vi "VisualizeCHROMAOUT.vi"() -> ()   [LabVIEW 2018, in "Visualization.lvlib" / "VisualizeAcPwr.lvclass"]
doc: "This VI listens for any measurement data associated with the provided PluginName and displays it to the user for analysis. The display is only suitable for data coming from the Chroma Plugin."
uses:
  VisualizeAcPwr.lvclass
  VisualizeBase/VisualizeBase_class/Requests/VisUserEventType.ctl
  <vilib>/event_ctls.llb/usereventprio.ctl
  AcPwr/AcPwrShared/clMeasurmentData.ctl
  <extravilib>/ChannelInstances/Tag-bool/Read With Abort.vi
  <extravilib>/ChannelInstances/Tag-bool/Write With Abort.vi
  <extravilib>/ChannelInstances/Tag-bool/Instantiate.vi
  <extravilib>/ChannelInstances/Tag-bool/EndpointRead.vi
  <vilib>/Utility/error.llb/Error Cluster From Error Code.vi
  <extravilib>/ChannelInstances/Tag-bool/Endpoint.vi
  <vilib>/ErrorRing/Error Ring.xnode
  VisualizeBase/VisualizeBase_class/VisualizeBase.lvclass
  <userlib>/NIST/NISTErrorLib/NISTErrorLib.lvlib
  AcPwr/AcPwrShared/AcPwrShared.lvlib
  <extravilib>/ChannelInstances/Tag-bool.lvlib
panel:
  in  "Tab Control":enum32{"Chart", "XY Graph"}(tab)
  out "ChromaOutput":waveform(dbl)[](graph)=[{"t0"=timestamp(3657200531.6397257 s since 1904-01-01), "dt"=1.0, "Y"=[46.19]}, {"t0"=timestamp(3657200531.6397257 s since 1904-01-01), "dt"=1.0, "Y"=[2.0]}, {"t0"=timestamp(3657200531.6397257 s since 1904-01-01), "dt"=1.0, "Y"=[60.0]}]
  in  "PlotYAxis":u32[](array[numeric])=[0, 1, 0] max=1
  out "Incorrect DataType?":bool
  out "Chroma's Internal Errors/Warnings":string="No Error"
  out "Current (A)":dbl(knob) scale=0.0..15.0
  out "Voltage (V)":dbl(knob) scale=0.0..100.0
  out "XY Graph":cluster{dbl[], dbl[]}(graph)={[0.02, 0.02, 0.02, 0.02, 0.02, 0.02, 0.02, 0.02, 0.1, 0.1, 0.1, 0.1, 0.1, 0.11, 0.2, 0.2, 0.2, 0.2, 0.2, 0.2, 0.3, 0.3, 0.3, 0.3, 0.3, 0.3, 0.3, 0.37, 0.4, 0.4, 0.4, 0.4, 0.4, 0.4, 0.48, 0.5, 0.5, 0.5, 0.5, 0.5, 0.5, 0.59, 0.6, 0.6, 0.6, 0.6, 0.6, 0.6, 0.6, 0.69, 0.69, 0.69, 0.69, 0.69, 0.69, 0.71, 0.79, 0.79, 0.79, 0.79, 0.79, 0.79, 0.89, 0.89, 0.89, 0.89, 0.89, 0.89, 0.89, 1.0, 1.0, 1.0, 1.0, 1.0, 1.0, 1.0, 1.1, 1.1, 1.1, 1.09, 1.09, 1.09, 1.1, 1.19, 1.19, 1.2, 1.2, 1.2, 1.2, 1.2, 1.29, 1.29, 1.29, 1.29, 1.29, 1.29, 1.29, 1.39, 1.39, 1.39, 1.39, 1.39, 1.39, 1.39, 1.4, 1.49, 1.49, 1.49, 1.49, 1.49, 1.49, 1.57, 1.59, 1.59, 1.59, 1.59, 1.59, 1.59, 1.69, 1.69, 1.69, 1.69, 1.69, 1.69, 1.69, 1.79, 1.79, 1.79, 1.79, 1.79, 1.79, 1.79, 1.89, 1.89, 1.89, 1.89, 1.89, 1.89, 1.89, 1.99, 1.99, 1.99, 1.99, 1.99, 1.99, 2.0, 2.09, 2.09, 2.09, 2.09, 2.09, 2.09, 2.13, 2.19, 2.19, 2.19, 2.19, 2.19, 2.19, 2.29, 2.29, 2.29, 2.29, 2.29, 2.29, 2.29, 2.29, 2.39, 2.39, 2.39, 2.39, 2.39, 2.39, 2.39, 2.49, 2.49, 2.49, 2.49, 2.49, 2.49, 2.51, 2.59, 2.59, 2.59, 2.59, 2.59, 2.59, 2.69, 2.69, 2.69, 2.69, 2.69, 2.69, 2.69, 2.79, 2.79, 2.79, 2.79, 2.79, 2.79, 2.79, 2.81, 2.89, 2.89, 2.89, 2.89, 2.89, 2.89, 2.89, 2.99, 2.99, 2.99, 2.99, 2.99, 2.99, 3.0, 3.09, 3.09, 3.09, 3.09, 3.09, 3.09, 3.1, 3.19, 3.19, 3.19, 3.19, 3.19, 3.19, 3.29, 3.29, 3.29, 3.29, 3.29, 3.29, 3.29, 3.39, 3.39, 3.39, 3.39, 3.39, 3.39, 3.39, 3.39, 3.49, 3.49, 3.49, 3.49, 3.49, 3.49, 3.49, 3.5, 3.59, 3.59, 3.59, 3.59, 3.59, 3.59, 3.6, 3.69, 3.69, 3.69, 3.69, 3.69, 3.69, 3.79, 3.79, 3.79, 3.79, 3.79, 3.79, 3.79, 3.89, 3.89, 3.89, 3.89, 3.89, 3.89, 3.89, 3.99, 3.99, 3.99, 3.99, 3.99, 3.99, 3.99], [42.02, 41.83, 42.15, 41.98, 41.52, 41.47, 41.64, 41.55, 41.51, 41.49, 41.46, 41.51, 41.41, 41.39, 41.42, 41.42, 41.41, 41.4, 41.29, 41.3, 41.32, 41.33, 41.32, 41.31, 41.32, 41.21, 41.21, 41.2, 41.2, 41.21, 41.22, 41.21, 41.1, 41.1, 41.09, 41.1, 41.09, 41.11, 41.1, 40.98, 40.99, 40.98, 40.98, 40.99, 40.99, 40.98, 40.98, 40.86, 40.86, 40.88, 40.87, 40.88, 40.87, 40.87, 40.74, 40.75, 40.75, 40.75, 40.73, 40.76, 40.63, 40.63, 40.62, 40.64, 40.64, 40.61, 40.64, 40.6, 40.5, 40.46, 40.5, 40.51, 40.5, 40.51, 40.37, 40.37, 40.37, 40.37, 40.37, 40.38, 40.37, 40.36, 40.22, 40.23, 40.23, 40.24, 40.23, 40.24, 40.1, 40.09, 40.07, 40.11, 40.09, 40.09, 40.11, 39.96, 39.96, 39.95, 39.96, 39.96, 39.96, 39.94, 39.81, 39.79, 39.79, 39.81, 39.8, 39.79, 39.79, 39.81, 39.65, 39.65, 39.65, 39.65, 39.64, 39.64, 39.65, 39.48, 39.48, 39.48, 39.48, 39.47, 39.48, 39.31, 39.31, 39.3, 39.31, 39.32, 39.31, 39.31, 39.14, 39.13, 39.13, 39.14, 39.13, 39.14, 39.13, 38.95, 38.95, 38.95, 38.94, 38.95, 38.95, 38.95, 38.75, 38.75, 38.76, 38.76, 38.75, 38.75, 38.75, 38.56, 38.56, 38.56, 38.56, 38.56, 38.55, 38.34, 38.34, 38.34, 38.33, 38.33, 38.34, 38.34, 38.11, 38.11, 38.1, 38.11, 38.12, 38.1, 38.11, 38.11, 37.87, 37.86, 37.86, 37.88, 37.86, 37.88, 37.86, 37.6, 37.61, 37.61, 37.61, 37.61, 37.61, 37.62, 37.33, 37.34, 37.33, 37.34, 37.34, 37.34, 37.04, 37.04, 37.05, 37.04, 37.06, 37.05, 37.04, 36.72, 36.72, 36.71, 36.72, 36.73, 36.72, 36.71, 36.72, 36.38, 36.37, 36.39, 36.37, 36.37, 36.38, 36.37, 36.0, 36.0, 35.99, 36.0, 35.99, 36.0, 35.99, 35.59, 35.59, 35.58, 35.58, 35.58, 35.58, 35.12, 35.12, 35.12, 35.13, 35.13, 35.13, 35.12, 34.6, 34.59, 34.59, 34.59, 34.59, 34.59, 34.59, 34.6, 33.97, 33.97, 33.98, 33.97, 33.98, 33.98, 33.98, 33.26, 33.27, 33.26, 33.26, 33.26, 33.26, 33.26, 33.26, 32.38, 32.39, 32.39, 32.37, 32.37, 32.39, 32.38, 31.25, 31.24, 31.25, 31.25, 31.25, 31.25, 29.64, 29.66, 29.66, 29.67, 29.65, 29.66, 29.66, 27.14, 27.15, 27.15, 27.15, 27.14, 27.14, 27.15, 17.86, 17.84]}
  in  "PluginName":string="AcPwr.ChromaPowerSupply0"
  out "ErrorArray":errorcluster[](array[cluster])
  in  "btnStop":bool
  in  "btnReset":bool
  in  "btnClear":bool
  # "0=Left Axis and 1=Right Axis"
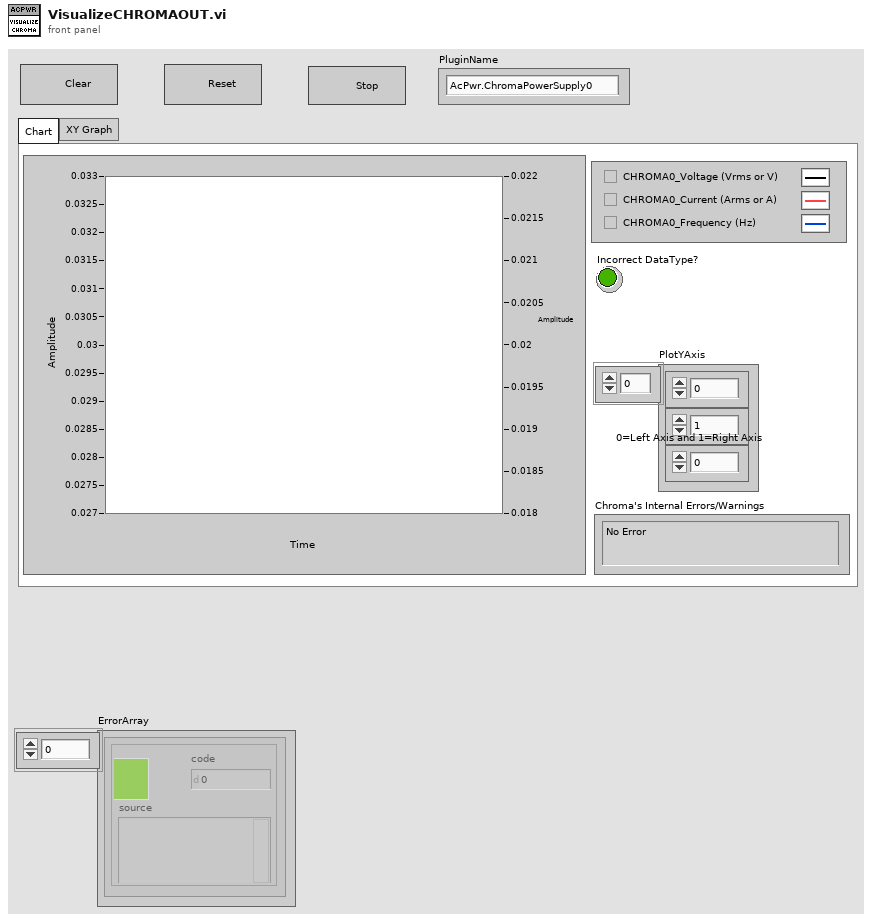
[diagram p1: front panel]
types:
  T1 = typedef "Visualization.lvlib/VisualizeBase.lvclass/VisRequestEvents.ctl" = cluster{"StopRequest":refnum<user-event>, "ResetRequest":refnum<user-event>, "FP Pop In or Out":refnum<user-event>}
  T2 = typedef "AcPwrShared.lvlib/AcPwrBroadcastEvents.ctl" = cluster{"DidInit":refnum<user-event>, "StatusUpdate":refnum<user-event>, "ErrorReport":refnum<user-event>, "DidStop":refnum<user-event>, "PathToINI":refnum<user-event>, "Measurements":refnum<user-event>, "LoadConfigFile":refnum<user-event>, "GetSettings":refnum<user-event>, "SetSettings":refnum<user-event>, "GetType&ID":refnum<user-event>, "GotSettings":refnum<user-event>}
  T3 = typedef "AcPwrShared.lvlib/clMeasurmentData.ctl" = cluster{"MeasName":string, "XML Data":string, "WaveformData":waveform(dbl)[]}
  T4 = typedef "Visualization.lvlib/VisualizeBase.lvclass/VisUserEventType.ctl" = cluster{"BusIndex":i8, "Data":variant}
  T5 = typedef "usereventprio.ctl" = enum32{"high priority", "normal priority"}
  T6 = typedef "Tag-bool.lvlib/))Channel.ctl" = refnum<queue>
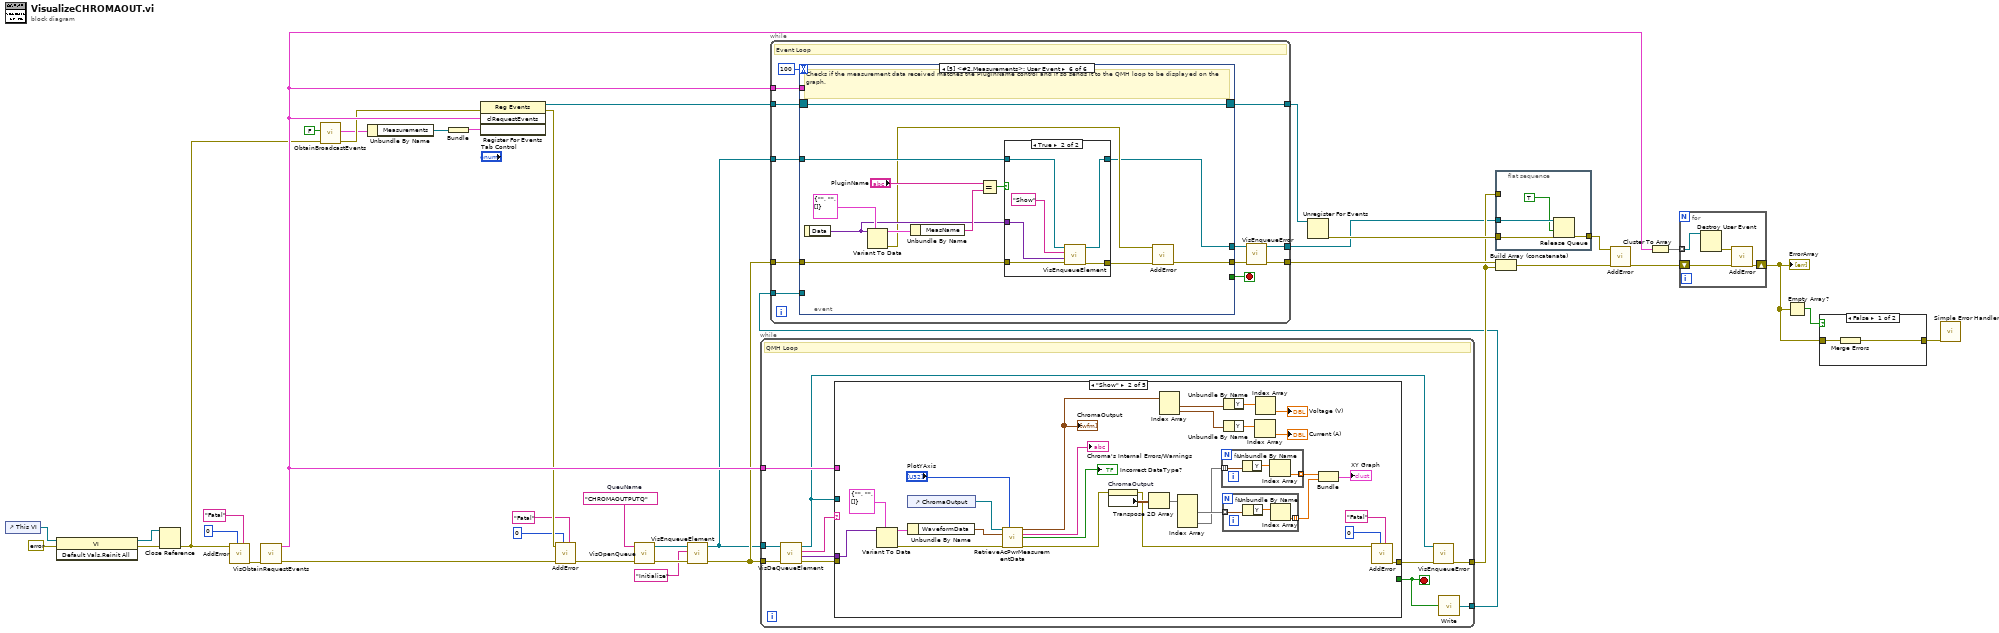
[diagram p0: block diagram]
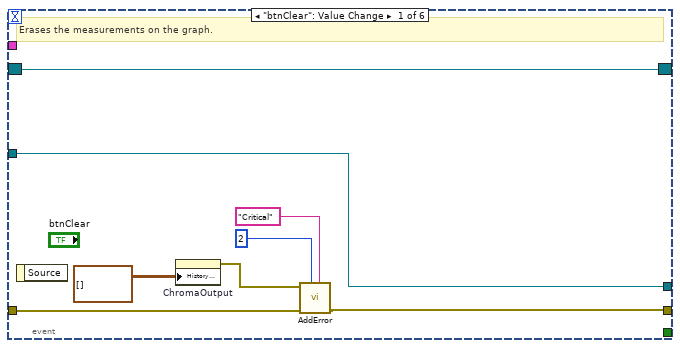
[diagram p2: hidden frame]
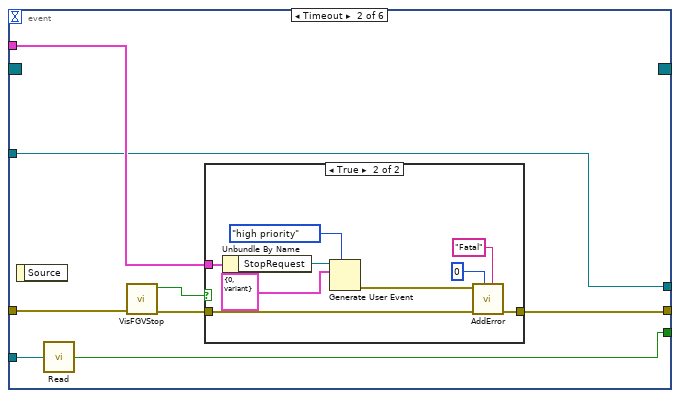
[diagram p3: hidden frame]
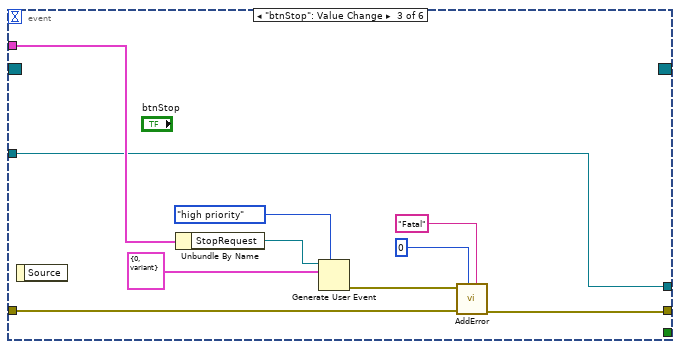
[diagram p5: hidden frame]
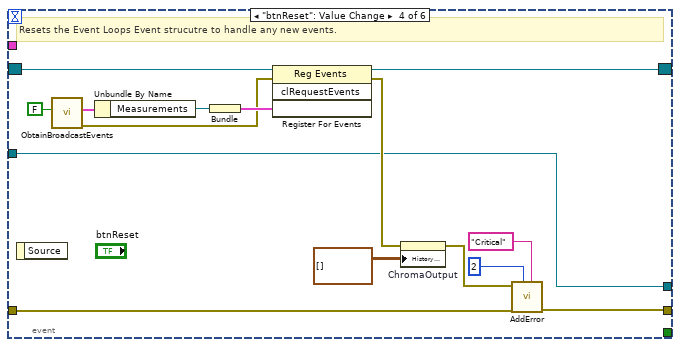
[diagram p6: hidden frame]
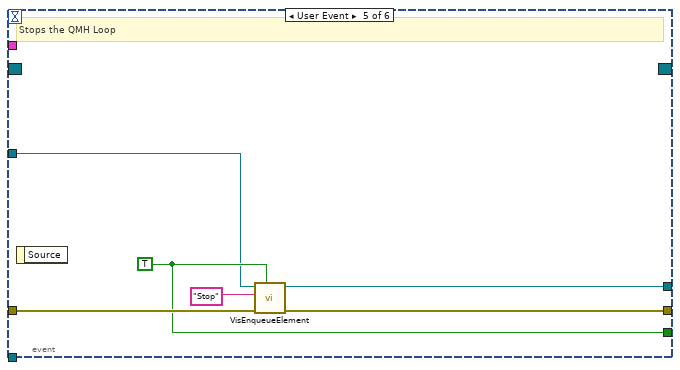
[diagram p7: hidden frame]
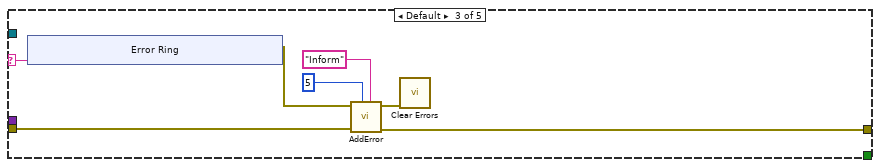
[diagram p10: hidden frame]
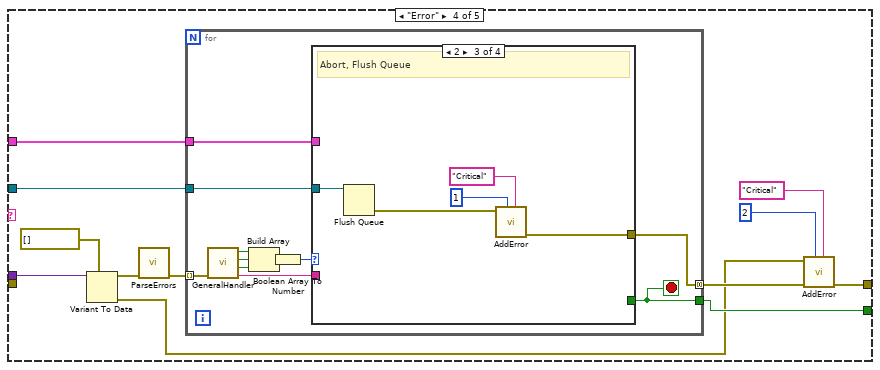
[diagram p11: hidden frame]
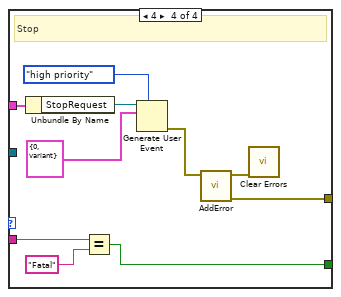
[diagram p14: hidden frame]
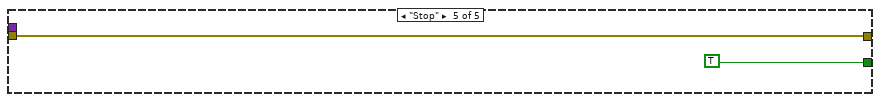
[diagram p15: hidden frame]
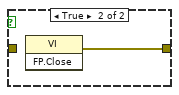
[diagram p16: hidden frame]
diagram:
  w10 = "CHROMAOUTPUTQ"  # QueuName
  n1 = control-ref of="This VI"() -> (w26:refnum<vi>)
  n2 = invoke class="VI" method="Default Vals.Reinit All"(reference=w26, error in=errorcluster {"status"=FALSE, "code"=0, "source"=""} ("error in (no error)")) -> (reference out=w23:refnum<vi>, error out=w24:errorcluster)  [unwired: 1 in, 1 out]
  n3 = Close Reference(reference=w23, error in (no error)=w24) -> (error out=w14:errorcluster)
  n4 = call <userlib>:"AddError.vi"("Severity"="Fatal", "Priority"=u8 0, "error in (no error)"=w14) -> ("ErrorArray Out"=w38:errorcluster[])  [unwired: 7 in, 1 out]
  n5 = call "VisObtainRequestEvents.vi"("Error"=w38) -> ("Error"=w21:errorcluster[], "clRequestEvents"=w30:T1)  [unwired: 9 in]
  n6 = call "ObtainBroadcastEvents.vi"("error in (no error)"=w14, "CreateNew? (F)"=FALSE) -> ("error out"=w15:errorcluster, "clAcPwrEvents"=w13:T2)  [unwired: 8 in]
  n7 = Unbundle By Name(w13) -> ("Measurements"=w28:refnum<user-event>)
  n8 = Bundle("Measurements"=w28) -> (w27:cluster{"Measurements":refnum<user-event>})  [unwired: 1 in]
  n9 = register-events(error in=w15, w30, w27) -> (reference out=w39:refnum<event-registration>, error out=w19:errorcluster)  [unwired: 1 in]
  n10 = call <userlib>:"AddError.vi"("Severity"="Fatal", "Priority"=u8 0, "ErrorArray In"=w21, "error in (no error)"=w19) -> ("ErrorArray Out"=w11:errorcluster[])  [unwired: 6 in, 1 out]
  n11 = call "VisOpenQueue.vi"("Error Array In"=w11, "QueueName"=w10) -> ("Error Array Out"=w8:errorcluster[], "queue out"=w9:refnum<queue>)  [unwired: 8 in]
  n12 = call "VisEnqueueElement.vi"("Error Array In"=w8, "Message"="Initialize", "queue in"=w9) -> ("Error Array Out"=w6:errorcluster[], "queue out"=w5:refnum<queue>)  [unwired: 7 in]
  n13 = while {
    tunnel: w6 -> [w44]
    tunnel: [w47] -> w16
    tunnel: w5 -> [w43]
    tunnel: w30 -> [w49]
    tunnel: [w40] -> w1
    stop <- w50 stop-if-true
    # "QMH Loop"
    n14 = call "VisDeQueueElement.vi"("Error Array In"=w44, "Queue In"=w43) -> ("Error Array Out"=w42:errorcluster[], "Data"=w45:variant, "Message"=w46:string, "Queue Out"=w41:refnum<queue>)  [unwired: 6 in]
    n15 = case shown="\"Show\"" w46 {
      selector: w46 -> [_ _ w92 _ _]
      tunnel: w45 -> [_ w58 _ w111 _]
      tunnel: w42 -> [w51 _ w90 _ w138]
      tunnel: [w51 w79 w89 w101 w138] -> w48
      tunnel: [_ _ _ w107 TRUE] -> w50
      tunnel: w49 -> [_ _ _ w106 _]
      tunnel: w41 -> [_ _ _ w105 _]
      frame "Initialize" {
      }
      frame "Show" {
        n16 = Variant To Data(type=T3 {"MeasName"="", "XML Data"="", "WaveformData"=[]} ("MeasurmentDataCluster"), Variant=w58) -> (data=w56:T3, error out=w57:errorcluster)  [unwired: 1 in]
        n17 = control-ref of="ChromaOutput"() -> (w78:refnum<vi>)
        n18 = Unbundle By Name(w56) -> ("WaveformData"=w55:waveform(dbl)[])
        n19 = call "RetrieveAcPwrMeasurementData.vi"("WaveformChartReference"=w78, "PlotYScale"="PlotYAxis", "WaveformArrayIn"=w55, "error in (no error)"=w57) -> ("WaveformArrayOut"=w65:waveform(dbl)[], "OutputString(Chroma)"=→"Chroma's Internal Errors/Warnings":string, "Incorrect DataType?"=→"Incorrect DataType?":bool, "error out"=w73:errorcluster)  [unwired: 7 in, 1 out]
        "ChromaOutput" <- w65
        n20 = property on="ChromaOutput" class="WFChart (strict)"(error in=w73) -> (error out=w53:errorcluster, "History Data"=w71:waveform(dbl)[][])  [unwired: 1 in, 1 out]
        n21 = Transpose 2D Array(2D array=w71) -> (transposed array=w72:waveform(dbl)[][])
        n22 = Index Array(array=w65) -> (element #1=w64:waveform(dbl), element #2=w63:waveform(dbl))  [unwired: 2 in]
        n23 = Index Array(array=w72) -> (element #1=w68:waveform(dbl)[], element #2=w67:waveform(dbl)[])  [unwired: 4 in]
        n24 = for {
          tunnel: w67 -> [w85] mode=indexing
          tunnel: [w83] -> w69 mode=indexing
          n25 = Unbundle By Name(w85) -> ("Y"=w84:dbl[])
          n26 = Index Array(array=w84) -> (element=w83:dbl)  [unwired: 1 in]
        }
        n27 = for {
          tunnel: w68 -> [w82] mode=indexing
          tunnel: [w80] -> w70 mode=indexing
          n28 = Unbundle By Name(w82) -> ("Y"=w81:dbl[])
          n29 = Index Array(array=w81) -> (element=w80:dbl)  [unwired: 1 in]
        }
        n30 = Unbundle By Name(w64) -> ("Y"=w62:dbl[])
        n31 = Unbundle By Name(w63) -> ("Y"=w61:dbl[])
        n32 = Index Array(array=w61) -> (element=→"Current (A)":dbl)  [unwired: 1 in]
        n33 = Index Array(array=w62) -> (element=→"Voltage (V)":dbl)  [unwired: 1 in]
        n34 = Bundle(w69, w70) -> (→"XY Graph":cluster{dbl[], dbl[]})  [unwired: 1 in]
        n35 = call <userlib>:"AddError.vi"("Severity"="Fatal" ("String"), "Priority"=u8 0, "error in (no error)"=w53) -> ("ErrorArray Out"=w79:errorcluster[])  [unwired: 7 in, 1 out]
      }
      frame Default {
        n36 = xnode "Error Ring"("parameter 0"=w92) -> ("error out"=w91:errorcluster)
        n37 = call <userlib>:"AddError.vi"("Severity"="Inform" ("String"), "Priority"=u8 5, "ErrorArray In"=w90, "error in (no error)"=w91) -> ("ErrorArray Out"=w89:errorcluster[], "error out"=w88:errorcluster)  [unwired: 6 in]
        n38 = call <vilib>:"Clear Errors.vi"("error in (no error)"=w88) -> ()  [unwired: 5 in, 2 out]
      }
      frame "Error" {
        n39 = Variant To Data(type=errorcluster[] [], Variant=w111) -> (data=w109:errorcluster[], error out=w100:errorcluster)  [unwired: 1 in]
        n40 = call <userlib>:"ParseErrors.vi"("ErrorArray"=w109) -> ("ErrorArray"=w108:errorcluster[])  [unwired: 8 in, 2 out]
        n41 = for {
          tunnel: w108 -> [w122] mode=indexing
          tunnel: [w116] -> w102 mode=concatenating
          tunnel: [w114] -> w107
          tunnel: w106 -> [w113]
          tunnel: w105 -> [w112]
          stop <- w114 stop-if-true
          n42 = call <userlib>:"GeneralHandler.vi"("error in (no error)"=w122) -> ("Severity"=w115:string, "Stop"=w119:bool, "Abort"=w120:bool, "Continue"=w121:bool)  [unwired: 6 in, 1 out]
          n43 = Build Array(w121, w120, w119) -> (w118:bool[])
          n44 = Boolean Array To Number(Boolean array=w118) -> (number=w117:u32)
          n45 = case shown="2" w117 {
            tunnel: [_ _ w127 w136] -> w116
            tunnel: w115 -> [_ _ _ w129]
            tunnel: [_ _ _ w131] -> w114
            tunnel: w113 -> [_ _ _ w130]
            tunnel: w112 -> [_ _ w123 _]
            frame 0, Default {
              # "No Dialog"
            }
            frame 1 {
              # "Continue"
            }
            frame 2 {
              # "Abort, Flush Queue"
              n46 = Flush Queue(queue=w123) -> (error out=w126:errorcluster)  [unwired: 1 in, 2 out]
              n47 = call <userlib>:"AddError.vi"("Severity"="Critical" ("String"), "Priority"=u8 1, "error in (no error)"=w126) -> ("ErrorArray Out"=w127:errorcluster[])  [unwired: 7 in, 1 out]
            }
            frame 4 {
              # "Stop"
              n48 = Unbundle By Name(w130) -> ("StopRequest"=w137:refnum<user-event>)
              n49 = Equal?(x=w129, y="Fatal" ("x")) -> (x = y?=w131:bool)
              n50 = Generate User Event(priority (normal)=usereventprio."high priority", user event=w137, event data cluster=T4 {"BusIndex"=0, "Data"=variant} ("event data")) -> (error out=w135:errorcluster)  [unwired: 1 in, 1 out]
              n51 = call <userlib>:"AddError.vi"("error in (no error)"=w135) -> ("ErrorArray Out"=w136:errorcluster[], "error out"=w132:errorcluster)  [unwired: 9 in]
              n52 = call <vilib>:"Clear Errors.vi"("error in (no error)"=w132) -> ()  [unwired: 5 in, 2 out]
            }
          }
        }
        n53 = call <userlib>:"AddError.vi"("Severity"="Critical", "Priority"=u8 2, "ErrorArray In"=w102, "error in (no error)"=w100) -> ("ErrorArray Out"=w101:errorcluster[])  [unwired: 6 in, 1 out]
      }
      frame "Stop" {
      }
    }
    n54 = call "VisEnqueueError.vi"("Error Array In"=w48, "Queue in"=w41) -> ("Error Array Out"=w47:errorcluster[])  [unwired: 8 in, 1 out]
    n55 = call <extravilib>:"Write.vi"("element"=w50) -> ("channel"=w40:T6)  [unwired: 1 out]
  }
  n56 = while {
    tunnel: w39 -> [w151]
    tunnel: [w145] -> w35
    tunnel: [w149] -> w37
    tunnel: w30 -> [w148]
    tunnel: w6 -> [w147]
    tunnel: w5 -> [w146]
    tunnel: [w142] -> w4
    tunnel: w1 -> [w140]
    stop <- w150 stop-if-true
    # "Event Loop"
    n57 = event shown="[5] <#2.Measurements>: User Event" {
      selector: w151 -> [w153 _ _ w202 _ w209]
      dyn-events: [w153 _ _ w201 _ w209] -> w149
      timeout: 100 -> [_ _ _ _ _ _]
      tunnel: [_ w160 _ _ w205 _] -> w150
      tunnel: [w156 w162 w184 w197 w207 w213] -> w144
      tunnel: w148 -> [_ w164 w186 _ _ _]
      tunnel: w147 -> [w157 w165 w187 w198 w208 w219]
      tunnel: w146 -> [w152 w163 w185 w188 w203 w221]
      tunnel: [w152 w163 w185 w188 w206 w210] -> w143
      tunnel: w140 -> [_ w161 _ _ _ _]
      event "btnClear": Value Change {
        # "Erases the measurements on the graph."
        n58 = event-data() -> ()  [unwired: 1 in, 1 out]
        n59 = property on="ChromaOutput" class="WFChart (strict)"("History Data"=waveform(dbl)[][] []) -> (error out=w155:errorcluster)  [unwired: 2 in, 1 out]
        n60 = call <userlib>:"AddError.vi"("Severity"="Critical", "Priority"=u8 2, "ErrorArray In"=w157, "error in (no error)"=w155) -> ("ErrorArray Out"=w156:errorcluster[])  [unwired: 6 in, 1 out]
      }
      event Timeout {
        n61 = event-data() -> ()  [unwired: 1 in, 1 out]
        n62 = call <extravilib>:"Read.vi"("channel"=w161) -> ("element"=w160:bool)  [unwired: 1 in, 1 out]
        n63 = call "VisFGVStop.vi"("Error In"=w165) -> ("Error Out"=w166:errorcluster[], "Value"=w167:bool)  [unwired: 9 in]
        n64 = case shown="True" w167 {
          tunnel: w166 -> [w168 w177]
          tunnel: [w168 w170] -> w162
          tunnel: w164 -> [_ w169]
          frame False {
          }
          frame True {
            n65 = Unbundle By Name(w169) -> ("StopRequest"=w175:refnum<user-event>)
            n66 = Generate User Event(priority (normal)=usereventprio."high priority", user event=w175, event data cluster=T4 {"BusIndex"=0, "Data"=variant} ("event data")) -> (error out=w176:errorcluster)  [unwired: 1 in, 1 out]
            n67 = call <userlib>:"AddError.vi"("Severity"="Fatal" ("String"), "Priority"=u8 0, "ErrorArray In"=w177, "error in (no error)"=w176) -> ("ErrorArray Out"=w170:errorcluster[])  [unwired: 6 in, 1 out]
          }
        }
      }
      event "btnStop": Value Change {
        n68 = event-data() -> ()  [unwired: 1 in, 1 out]
        n69 = Unbundle By Name(w186) -> ("StopRequest"=w182:refnum<user-event>)
        n70 = Generate User Event(priority (normal)=usereventprio."high priority", user event=w182, event data cluster=T4 {"BusIndex"=0, "Data"=variant} ("event data")) -> (error out=w183:errorcluster)  [unwired: 1 in, 1 out]
        n71 = call <userlib>:"AddError.vi"("Severity"="Fatal" ("String"), "Priority"=u8 0, "ErrorArray In"=w187, "error in (no error)"=w183) -> ("ErrorArray Out"=w184:errorcluster[])  [unwired: 6 in, 1 out]
      }
      event "btnReset": Value Change {
        # "Resets the Event Loops Event strucutre to handle any new events."
        n72 = event-data() -> ()  [unwired: 1 in, 1 out]
        n73 = call "ObtainBroadcastEvents.vi"("CreateNew? (F)"=FALSE) -> ("error out"=w191:errorcluster, "clAcPwrEvents"=w190:T2)  [unwired: 9 in]
        n74 = Unbundle By Name(w190) -> ("Measurements"=w200:refnum<user-event>)
        n75 = Bundle("Measurements"=w200) -> (w199:cluster{"Measurements":refnum<user-event>})  [unwired: 1 in]
        n76 = register-events(reference=w202, error in=w191, w199) -> (reference out=w201:refnum<event-registration>, error out=w193:errorcluster)  [unwired: 1 in]
        n77 = property on="ChromaOutput" class="WFChart (strict)"(error in=w193, "History Data"=waveform(dbl)[][] []) -> (error out=w192:errorcluster)  [unwired: 1 in, 1 out]
        n78 = call <userlib>:"AddError.vi"("Severity"="Critical", "Priority"=u8 2, "ErrorArray In"=w198, "error in (no error)"=w192) -> ("ErrorArray Out"=w197:errorcluster[])  [unwired: 6 in, 1 out]
      }
      event User Event {
        w205 = TRUE ("Priority? (F)")
        # "Stops the QMH Loop"
        n79 = event-data() -> ()  [unwired: 1 in, 1 out]
        n80 = call "VisEnqueueElement.vi"("Priority? (F)"=w205, "Error Array In"=w208, "Message"="Stop", "queue in"=w203) -> ("Error Array Out"=w207:errorcluster[], "queue out"=w206:refnum<queue>)  [unwired: 6 in]
      }
      event User Event {
        # "Checks if the measurement data received matches the PluginName control and if so sends it to the QMH loop to be displayed on the graph."
        n81 = event-data() -> ("Data"=w214:variant)  [unwired: 1 in]
        n82 = Variant To Data(type=T3 {"MeasName"="", "XML Data"="", "WaveformData"=[]} ("MeasurmentDataCluster"), Variant=w214) -> (data=w216:T3, error out=w211:errorcluster)  [unwired: 1 in]
        n83 = Unbundle By Name(w216) -> ("MeasName"=w215:string)
        n84 = Equal?(x="PluginName", y=w215) -> (x = y?=w220:bool)
        n85 = case shown="True" w220 {
          tunnel: [w222 w228] -> w212
          tunnel: w221 -> [w223 w227]
          tunnel: w219 -> [w222 w229]
          tunnel: [w223 w225] -> w210
          tunnel: w214 -> [_ w226]
          frame False {
          }
          frame True {
            n86 = call "VisEnqueueElement.vi"("Error Array In"=w229, "Data"=w226, "Message"="Show", "queue in"=w227) -> ("Error Array Out"=w228:errorcluster[], "queue out"=w225:refnum<queue>)  [unwired: 6 in]
          }
        }
        n87 = call <userlib>:"AddError.vi"("ErrorArray In"=w212, "error in (no error)"=w211) -> ("ErrorArray Out"=w213:errorcluster[])  [unwired: 8 in, 1 out]
      }
    }
    n88 = call "VisEnqueueError.vi"("Error Array In"=w144, "Queue in"=w143) -> ("Error Array Out"=w145:errorcluster[], "Queue out"=w142:refnum<queue>)  [unwired: 8 in]
  }
  n89 = Unregister For Events(event registration refnum=w37) -> (error out=w34:errorcluster)  [unwired: 1 in]
  n90 = flat-sequence {
    tunnel: w34 -> [w233]
    tunnel: [w232] -> w32
    tunnel: w4 -> [w231]
    tunnel: w16 -> [_]
    frame #0 {
      n91 = Release Queue(queue=w231, force destroy? (F)=TRUE, error in (no error)=w233) -> (error out=w232:errorcluster)  [unwired: 2 out]
    }
  }
  n92 = Build Array (concatenate)(w35, w16) -> (w33:errorcluster[])
  n93 = call <userlib>:"AddError.vi"("ErrorArray In"=w33, "error in (no error)"=w32) -> ("ErrorArray Out"=w31:errorcluster[])  [unwired: 8 in, 1 out]
  n94 = Cluster To Array(cluster=w30) -> (array=w36:refnum<user-event>[])
  n95 = for {
    tunnel: w36 -> [w237] mode=indexing
    shift-right: [w236] -> w3
    shift-left: w31 -> [w235]
    n96 = Destroy User Event(user event=w237) -> (error out=w234:errorcluster)  [unwired: 1 in]
    n97 = call <userlib>:"AddError.vi"("ErrorArray In"=w235, "error in (no error)"=w234) -> ("ErrorArray Out"=w236:errorcluster[])  [unwired: 8 in, 1 out]
  }
  "ErrorArray" <- w3
  n98 = Empty Array?(array=w3) -> (empty?=w29:bool)
  n99 = case shown="False" w29 {
    tunnel: [w238 w240] -> w2
    tunnel: w3 -> [w239 _]
    frame False {
      n100 = Merge Errors(w239) -> (w238:errorcluster)
    }
    frame True {
      n101 = invoke class="VI" method="FP.Close"() -> (error out=w240:errorcluster)  [unwired: 3 in, 2 out]
    }
  }
  n102 = call <vilib>:"Simple Error Handler.vi"("error in (no error)"=w2) -> ()  [unwired: 4 in, 5 out]
